vi "RT Main v1.9.vi"() -> ()   [LabVIEW 2021]
doc: "Changelog:\n\nv1.9:\n- Added a new shift register for \"clean resume\" which is reset when starting autocycle, and when performing a homing. It is set always after completing autocycle.\n\nv0.9:\n- Autocycle"
uses:
  Controls/Auto Delays.ctl
  Controls/DO 1.ctl
  Controls/Modbus Input.ctl
  support/Controls/General Para.ctl
  support/Controls/All Inputs.ctl
  Controls/DI 1.ctl
  Controls/DI 2.ctl
  support/Controls/Index Details.ctl
  support/Controls/Auto Stats.ctl
  Controls/Auto Times.ctl
  Global Variables/RT GV.vi
  support/Message Queue/Enqueue Message (Single).vi
  Global Variables/FPGA GV.vi
  <vilib>/Utility/error.llb/Error Cluster From Error Code.vi
  <vilib>/rvi/errors/niLvFpgaAdjustHostInterfaceError.vi
  Global Variables/Network Globals.vi
  <vilib>/FPGAPlugInAG/Dynamic/niLvFpga_Close_Dynamic.vi
  <vilib>/Modbus/master/Modbus Master.lvclass
  <vilib>/rvi/interface/nirviReadWriteControl/nirviReadWriteControl.xnode
  <vilib>/rvi/interface/nirviCloseFPGA/nirviCloseFPGA.xnode
  Controls/FPGA Ref.ctl
  support/Message Queue/Message Queue.lvlib
  NiFpgaLv.dll
  <vilib>/rvi/interface/Simulation/niFpgaSimulationCallBeginRW.vi
panel:
  in  "Auto Para":T1={"Agitator Delays"=[250, 350], "TF Delays"=[700, 800, 2], "Insertion Delays"=[100, 500], "Cutting Delays"=[300, 300, 100], "PF Delays"=[250, 30000], "Measur. Delays"=[500.0, 188.9, 1.0], "Reject Delays"=[500], "BF Delays"=[1000, 1000], "P&P Delays"=[1000]}
  in  "Stop Button 4":bool
  out "error out":errorcluster
  out "Wrong Message":string
  in  "Stop Button":bool
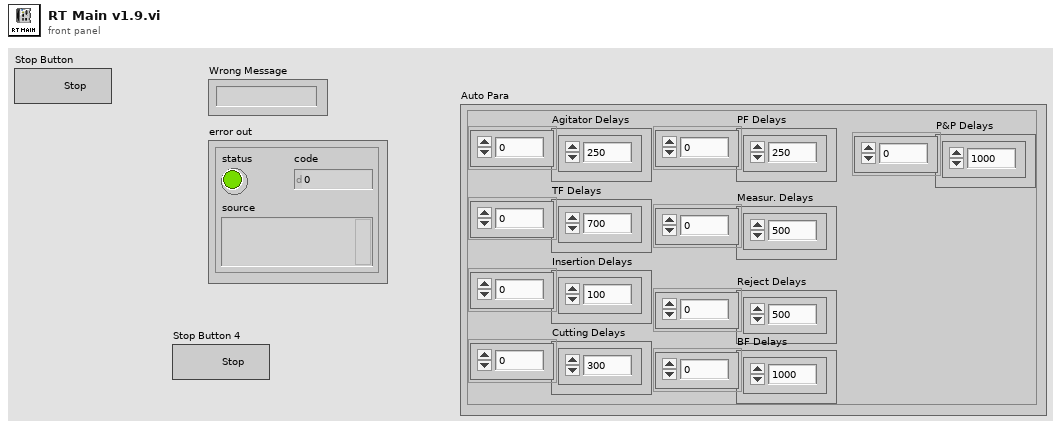
[diagram p1: front panel]
types:
  T1 = typedef "Auto Delays.ctl" = cluster{"Agitator Delays":u32[], "TF Delays":u32[], "Insertion Delays":u32[], "Cutting Delays":u32[], "PF Delays":u32[], "Measur. Delays":dbl[], "Reject Delays":u32[], "BF Delays":u32[], "P&P Delays":u32[]}
  T2 = typedef "FPGA Ref.ctl" = refnum<k20>
  T3 = typedef "DO 1.ctl" = cluster{"TL_Red":bool, "TL_Orange":bool, "TL_Green":bool, "TL_Buzzer":bool, "Vaccuum ON":bool, "Vaccuum OFF":bool, "Beckhoff Data":bool, "SOL_Singling":bool, "Bowl  Feeder_ ON 1":bool, "Buffer":bool, "SOL_Pick_Place_Vertical":bool, "SOL_Tube_Feed_Agitatator":bool, "SOL_Tube_Feed_Gating_CYL":bool, "SOL_Insertion _CYL":bool, "SOL_Insertion_Clamp_CYL":bool, "SOL_Cutting_CYL":bool, "SOL_Cutting_Clamp_CYL":bool, "SOL_Cutting_Foward_CYL":bool, "SOL_Measurement_CYL":bool, "SOL_Pick_Place_Rotary":bool, "SOL_Rejection CYL_1":bool, "SOL_Rejection CYL_2":bool, "SOL_Rejection CYL_3":bool, "SOL_Rejection CYL_4":bool, "Bowl  Feeder_ ON 2":bool, "Linear_Feeder 1":bool, "Linear_Feeder 2":bool, "Buffer 2":bool, "Buffer 3":bool, "Buffer 4":bool, "Buffer 5":bool, "Buffer 6":bool}
  T4 = typedef "Modbus Input.ctl" = cluster{"Maintenance Mode":bool, "Servo ON":bool, "Start":bool, "Stop":bool, "Reset Fault":bool, "Position Mode":bool, "Velocity Mode":bool, "Index":bool, "Start Index":bool, "Home":bool, "Start":bool, "Maintenance Position":i32, "Maintenance Hardware Torque":u16, "Maintenance Software Torque":u16, "Index Timeout":i16, "Index Position":i32, "Index Hardware Torque Limit":u16, "Index Software Torque Limit":u16, "Homing Timeout":i16, "Prehoming Position":i32, "Prehoming Hardware Torque Limit":u16, "Prehoming Software Torque Limit":u16, "Homing Position":i32, "Homing Hardware Torque Limit":u16, "Homing Software Torque Limit":u16}
  T5 = typedef "General Para.ctl" = cluster{"Max. Cons.":dbl, "Offset 1":dbl, "Offset 2":dbl, "Offset 3":dbl, "Offset 4":dbl, "OutputPause":dbl, "RejectPause":dbl, "IndexTimeout":dbl}
  T6 = typedef "All Inputs.ctl" = cluster{"DI 1":T7, "DI 2":T8, "IAS 1":dbl, "IAS 2":dbl, "IAS 3":dbl, "IAS 4":dbl, "DO 1":T3}
  T7 = typedef "DI 1.ctl" = cluster{"Machine_ON":bool, "E_stop ":bool, "SW_Pressure":bool, "SW_Start ":bool, "SW_Reset":bool, "SW_Stop":bool, "SW_Door":bool, "Buffer 1":bool, "Buffer 2":bool, "RS_Index_Stopper _Rear":bool, "RS_Singling_Rear":bool, "IPS_Index_Pallet_Sensor":bool, "PES_Index_Output_Part Sensor":bool, "Buffer 3":bool, "SW_Cutting_Station_Door":bool, "PES_BF_Pump_CNVR_Full_1":bool, "PES_BF_Pump_CNVR_Full_2":bool, "PES_BF_Pump_CNVR_Full_3":bool, "PES_BF_Pump_CNVR_Full_4":bool, "PES_PC_Pump Presence_1":bool, "PES_PC_Pump Presence_2":bool, "PES_PC_Pump Presence_3":bool, "PES_PC_Pump Presence_4":bool, "RS_Pick_Place_Vertical":bool, "Buffer 5":bool, "PES_TF_Low_Level":bool, "RS_Cutting_Rear1":bool, "RS_Cutting_Rear2":bool, "RS_Cutting_Rear3":bool, "RS_Cutting_Rear4":bool, "RS_Cutting_Forward_Rear":bool, "Buffer 11":bool}
  T8 = typedef "DI 2.ctl" = cluster{"RS_Agitatator_1_Rear":bool, "Buffer 1 ":bool, "RS_TF_Gating CYL_Rear":bool, "RS_Insertion_1_Rear":bool, "RS_Insertion_1_Front":bool, "RS_Insertion _2_Rear":bool, "RS_Insertion _2_Front":bool, "RS_Insertion _3_Rear":bool, "RS_Insertion _3_Front":bool, "RS_Insertion _4_Rear":bool, "RS_Insertion _4_Front":bool, "RS_Insertion_Clamp_CYL":bool, "RS_Cutting_Rear":bool, "RS_Clamping_Rear":bool, "RS_Measurement_Front":bool, "RS_Measurement_Rear":bool, "Buffer 2":bool, "Buffer 3":bool, "Buffer 4":bool, "RS_Rejection_1_Rear":bool, "RS_Rejection_2_Rear":bool, "RS_Rejection_3_Rear":bool, "RS_Rejection_4_Rear":bool, "Buffer 5":bool, "Buffer 6":bool, "LS_Rotary_P&P":bool, "Vaccum Components check":bool, "Buffer 9":bool, "Buffer 10":bool, "Buffer 11":bool, "Buffer 12":bool, "Buffer 13":bool}
  T9 = typedef "Index Details.ctl" = cluster{"Time (ms)":u32, "Waveform Graph":i16[]}
  T10 = cluster{T1, "Reject Pallets":cluster{"Reject 1":bool, "Reject 2":bool, "Reject 3":bool, "Reject 4":bool}}
  T11 = typedef "Auto Stats.ctl" = cluster{"Time-Stamp":timestamp, "Auto Times":T12, "Measurements":cluster{"1":dbl, "2":dbl, "3":dbl, "4":dbl}, "Outputs":cluster{"Good Parts":u32, "Reject Parts":u32}, "Cycle Time":dbl, "Remarks":string}
  T12 = typedef "Auto Times.ctl" = cluster{"Index Time":u32, "TF Time":u32, "Insertion Time":u32, "Cutting Time":u32, "PF Time":u32, "Meas. Time":u32, "Reject Time":u32, "P&P Time":u32}
  T13 = cluster{string, dbl, "cluster":cluster{"Auto Para":T1, "General Para":T5}}
  T14 = cluster{"TL_Red":bool, "TL_Orange":bool, "TL_Green":bool, "TL_Buzzer":bool, "Vaccuum ON":bool, "Vaccuum OFF":bool, "Beckhoff Data":bool, "SOL_Singling":bool, "Bowl Feeder_ ON1":bool, "Buffer 1":bool, "SOL_Pick_Place_Vertical":bool, "SOL_Tube_Feed_Agitatator":bool, "SOL_Tube_Feed_Gating_CYL":bool, "SOL_Insertion _CYL":bool, "SOL_Insertion_Clamp_CYL":bool, "SOL_Cutting_CYL":bool, "SOL_Cutting_Clamp_CYL":bool, "SOL_Insertion_Air_Nozzle":bool, "SOL_Measurement_CYL":bool, "SOL_Pick_Place_Rotary":bool, "SOL_Rejection CYL_1":bool, "SOL_Rejection CYL_2":bool, "SOL_Rejection CYL_3":bool, "SOL_Rejection CYL_4":bool, "Bowl Feeder_ON2":bool, "Linear Feeder 1":bool, "Linear Feeder 2":bool, "Buffer 2":bool, "Buffer 3":bool, "Buffer 4":bool, "Buffer 5":bool, "Buffer 6":bool}
  T15 = cluster{"Machine_ON":bool, "E_stop ":bool, "SW_Pressure":bool, "SW_Start ":bool, "SW_Reset":bool, "SW_Stop":bool, "SW_Door":bool, "Buffer 1":bool, "Buffer 2":bool, "RS_Index_Stopper _Rear":bool, "RS_Singling_Rear":bool, "PES_Index_Pallet_Sensor":bool, "PES_Index_Output_Part Sensor":bool, "Buffer 3":bool, "SW_Cutting_Station_Door":bool, "ICS_BF_Pump_CNVR_Full_1":bool, "ICS_BF_Pump_CNVR_Full_2":bool, "ICS_BF_Pump_CNVR_Full_3":bool, "ICS_BF_Pump_CNVR_Full_4":bool, "PES_PC_Pump Presence_1":bool, "PES_PC_Pump Presence_2":bool, "PES_PC_Pump Presence_3":bool, "PES_PC_Pump Presence_4":bool, "RS_Pick_Place_Vertical":bool, "Buffer 4":bool, "PES_TF_Low_Level":bool, "RS_Cutting_Rear 1":bool, "RS_Cutting_Rear 2":bool, "RS_Cutting_Rear 3":bool, "RS_Cutting_Rear 4":bool, "RS_Cutting_Forward_Rear":bool, "Buffer 10":bool}
  T16 = cluster{"RS_Agitatator_1_Rear ":bool, "Buffer 1 ":bool, "RS_TF_Gating CYL_Rear":bool, "RS_Insertion_1_Rear":bool, "RS_Insertion_1_Front":bool, "RS_Insertion _2_Rear":bool, "RS_Insertion _2_Front":bool, "RS_Insertion _3_Rear":bool, "RS_Insertion _3_Front":bool, "RS_Insertion _4_Rear":bool, "RS_Insertion _4_Front":bool, "RS_Insertion_Clamp_CYL":bool, "RS_Cutting_Rear":bool, "RS_Clamping_Rear":bool, "RS_Measurement_Front":bool, "RS_Measurement_Rear":bool, "Buffer 3":bool, "Buffer 4":bool, "Buffer 5":bool, "RS_Rejection_1_Rear":bool, "RS_Rejection_2_Rear":bool, "RS_Rejection_3_Rear":bool, "RS_Rejection_4_Rear":bool, "Buffer 6 ":bool, "Buffer 7 ":bool, "LS_Rotary_P&P":bool, "Vaccum Components check":bool, "Buffer 10 ":bool, "Buffer 11 ":bool, "Buffer 12 ":bool, "Buffer 13 ":bool, "Buffer 14":bool}
  T17 = cluster{"Array":string[][], "Machine Status":string}
  T18 = cluster{"Measurements":cluster{"1":dbl, "2":dbl, "3":dbl, "4":dbl}, "Reject Pallets":cluster{"Reject 1":bool, "Reject 2":bool, "Reject 3":bool, "Reject 4":bool}}
  T19 = cluster{"Auto Times":T12, "Results":cluster{"Measurements":cluster{"1":dbl, "2":dbl, "3":dbl, "4":dbl}, "Reject Pallets":cluster{"Reject 1":bool, "Reject 2":bool, "Reject 3":bool, "Reject 4":bool}}, "OutputCount":u32, "error out":errorcluster}
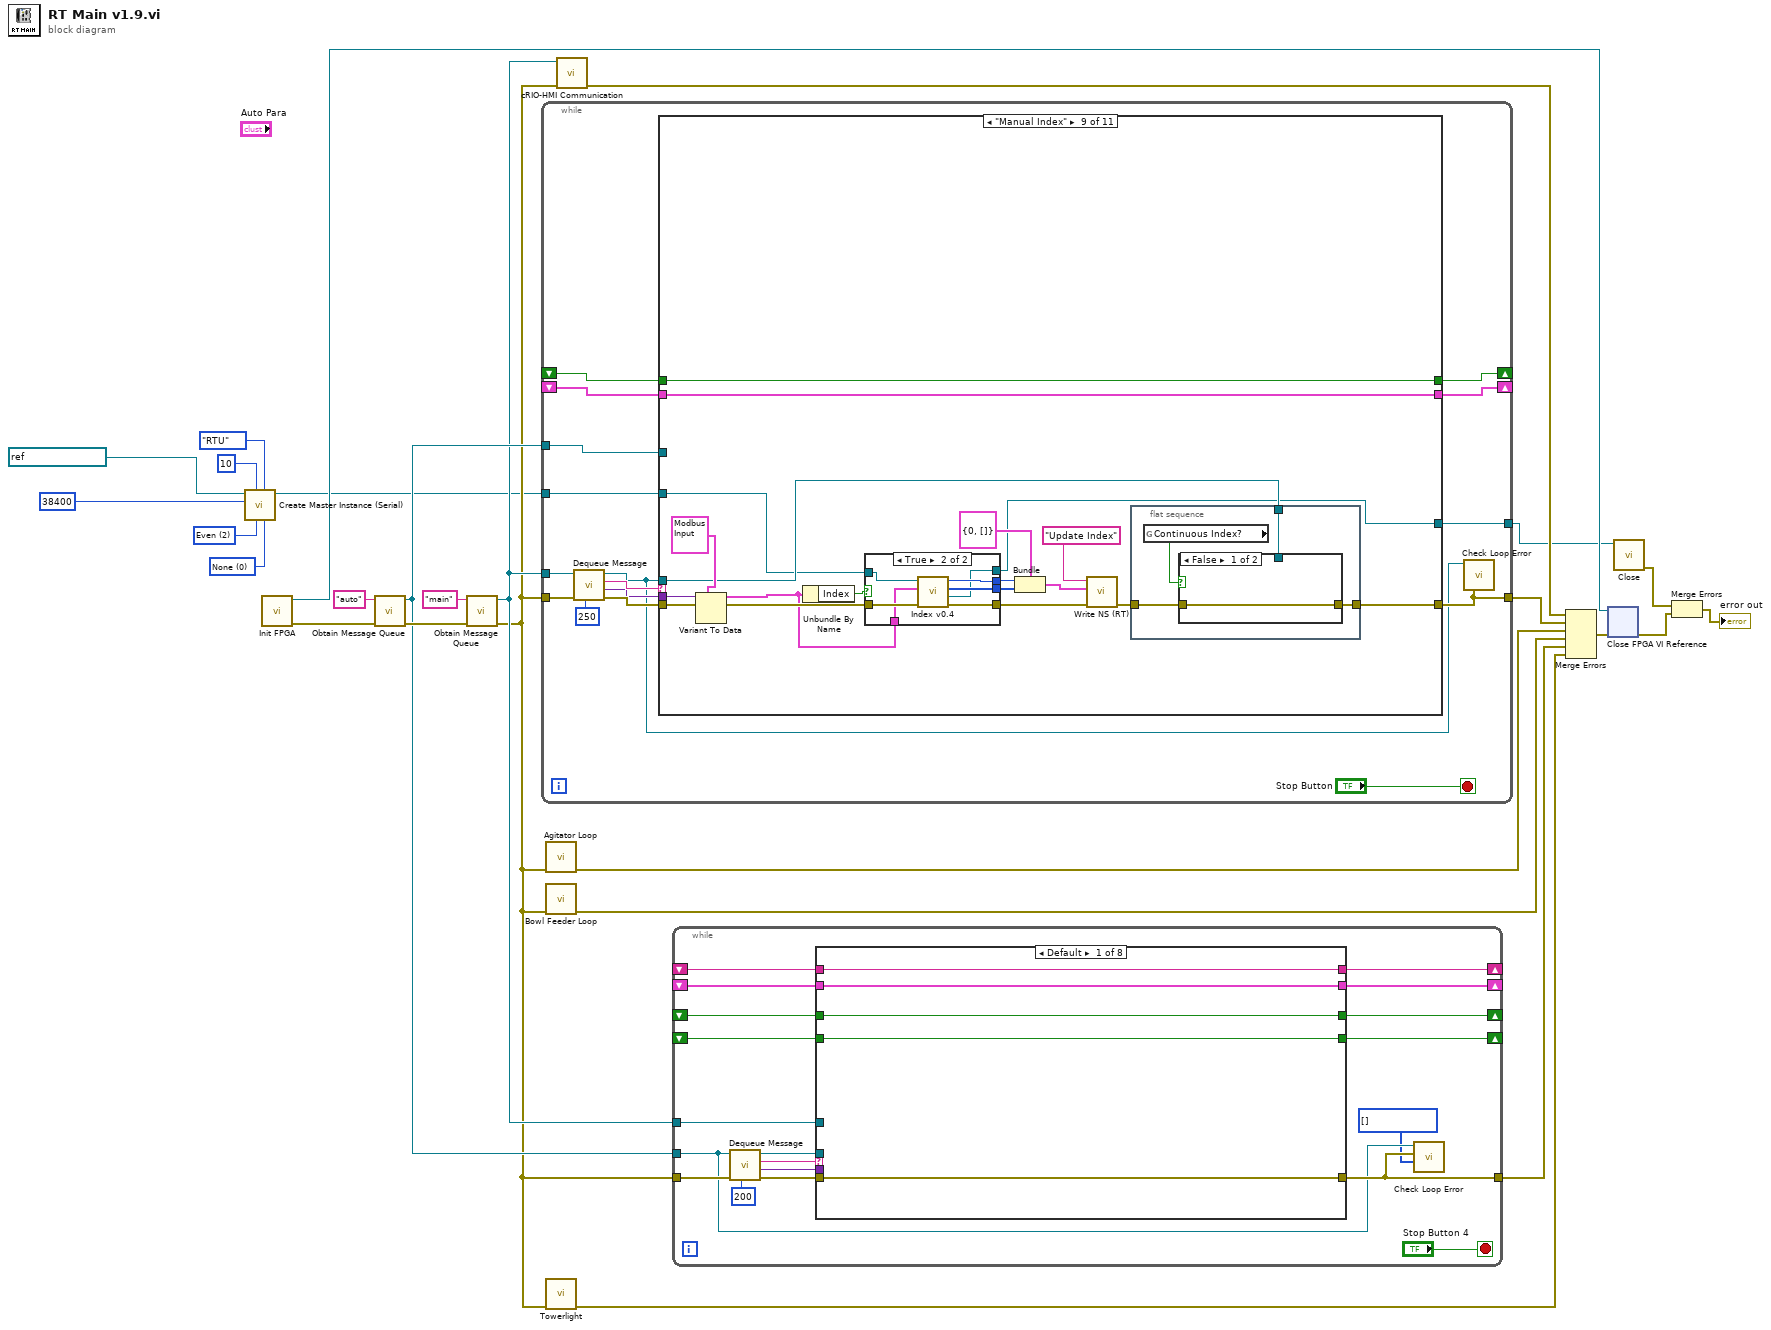
[diagram p0: block diagram]
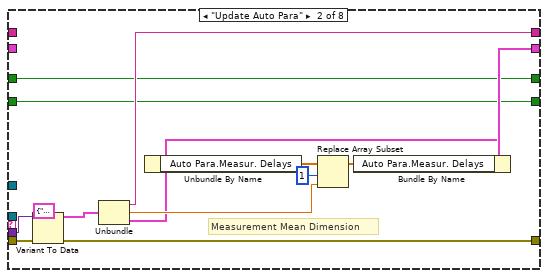
[diagram p2: hidden frame]
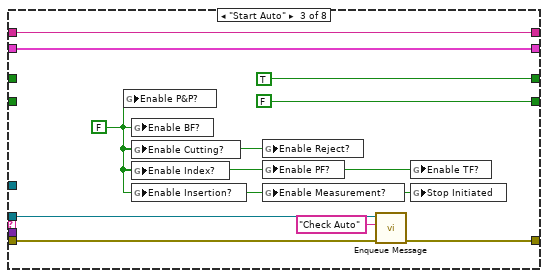
[diagram p3: hidden frame]
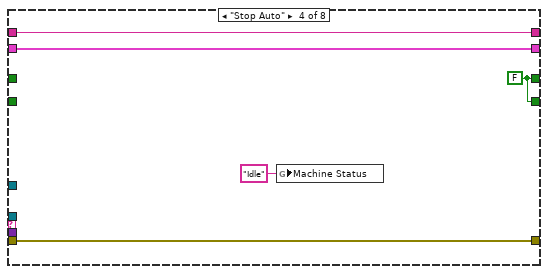
[diagram p4: hidden frame]
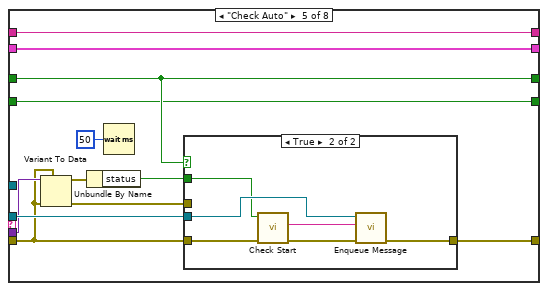
[diagram p5: hidden frame]
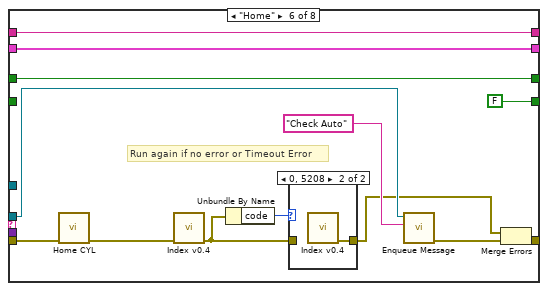
[diagram p7: hidden frame]
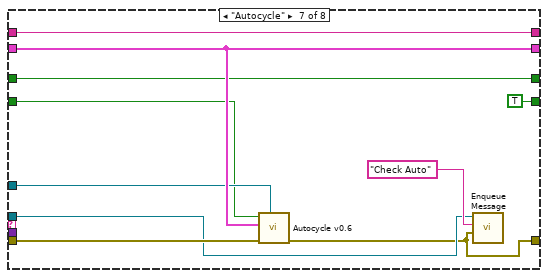
[diagram p9: hidden frame]
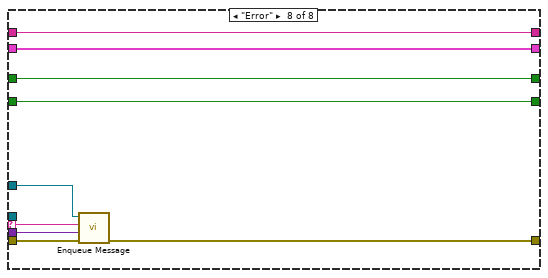
[diagram p10: hidden frame]
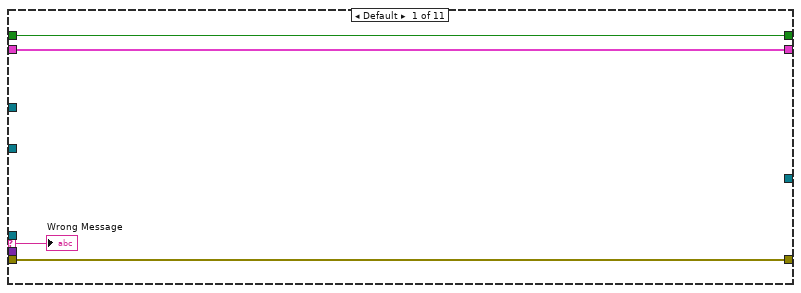
[diagram p11: hidden frame]
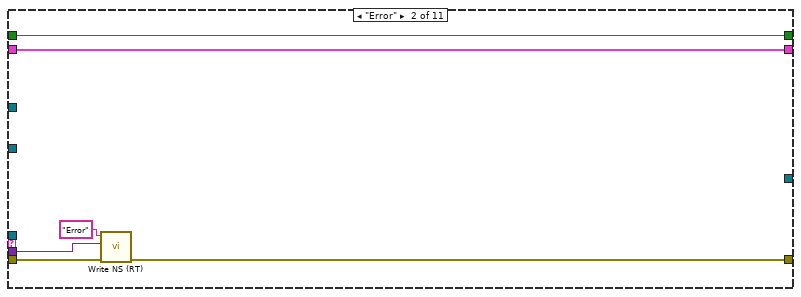
[diagram p12: hidden frame]
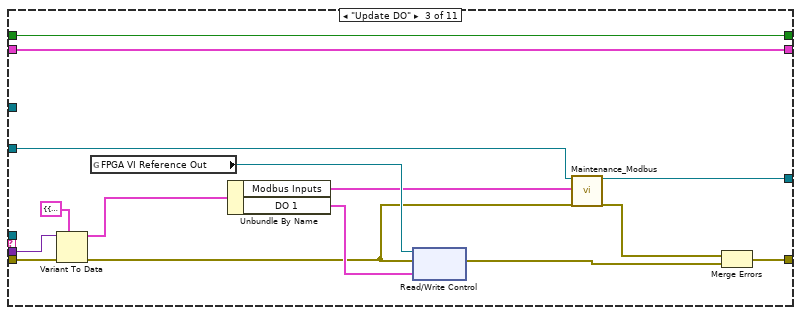
[diagram p13: hidden frame]
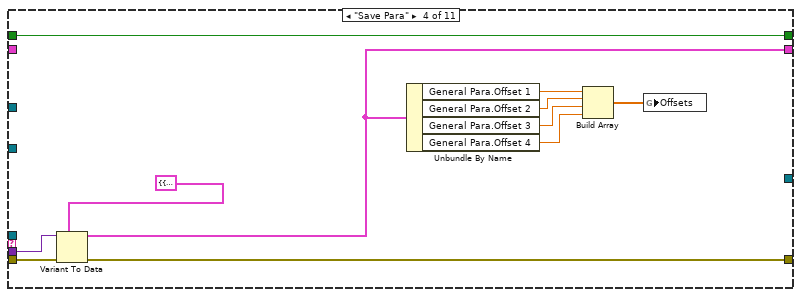
[diagram p14: hidden frame]
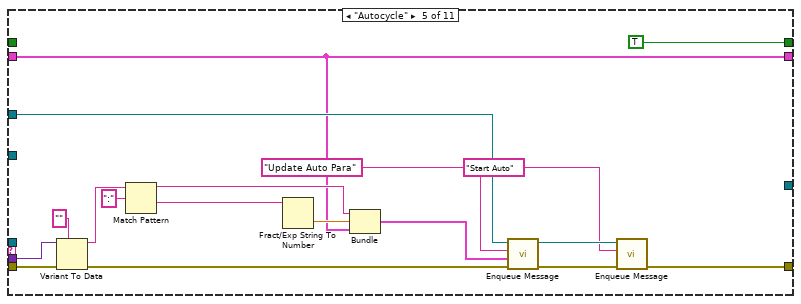
[diagram p15: hidden frame]
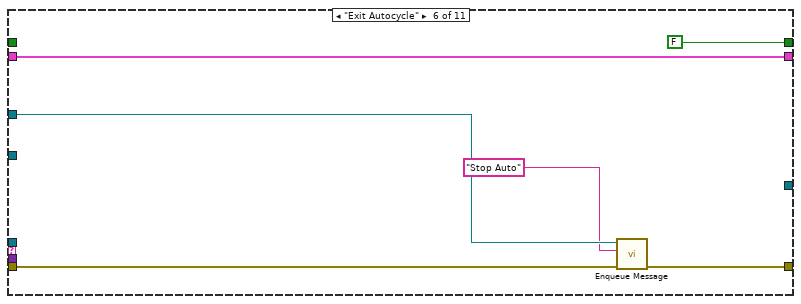
[diagram p16: hidden frame]
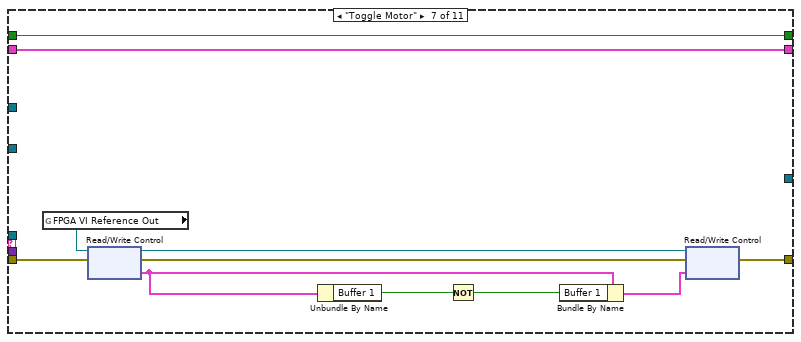
[diagram p17: hidden frame]
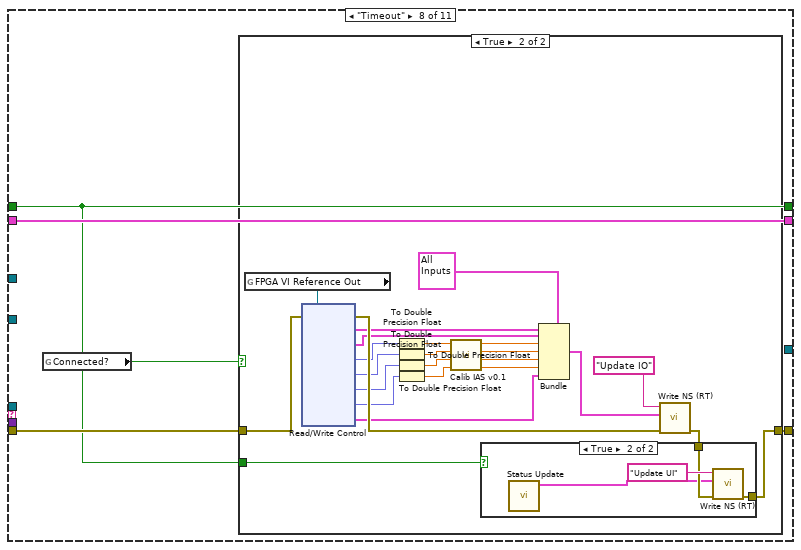
[diagram p18: hidden frame]
diagram:
  w6 = u16 0 items=["None", "XON/XOFF", "RTS/CTS", "XON/XOFF & RTS/CTS", "DTR/DSR", "XON/XOFF & DTR/DSR"] ("flow control (None)")
  w7 = u16 2 items=["None", "Odd", "Even"] ("parity (Even)")
  n1 = call <vilib>:"Create Master Instance (Serial).vi"("flow control (None)"=w6, "serial type"=enum16{"RTU", "ASCII"}."RTU", "parity (Even)"=w7, "unit ID"=u8 10, "baud rate (9600)"=u32 38400, "VISA resource name"=refnum<visa-resource-name> "ASRL1::INSTR") -> ("serial master instance"=w2:refnum<class "Modbus Master.lvclass">)  [unwired: 4 in, 1 out]
  n2 = call "Init FPGA.vi"() -> ("error out"=w17:errorcluster, "FPGA Ref Out"=w21:T2)  [unwired: 10 in]
  n3 = call "Obtain Message Queue.vi"("error in (no error)"=w17, "name"="auto") -> ("error out"=w16:errorcluster, "Message Queue"=w15:refnum<queue>)  [unwired: 8 in]
  n4 = call "Obtain Message Queue.vi"("error in (no error)"=w16, "name"="main") -> ("error out"=w13:errorcluster, "Message Queue"=w14:refnum<queue>)  [unwired: 8 in]
  n5 = while {
    tunnel: w13 -> [w41]
    tunnel: w14 -> [w40]
    tunnel: [w36] -> w26
    tunnel: w15 -> [w33]
    shift-right: [w31] -> _
    shift-left: _ -> [w32]
    shift-right: [w29] -> _
    shift-left: _ -> [w30]
    tunnel: w2 -> [w27]
    tunnel: [w28] -> w1
    stop <- "Stop Button" stop-if-true
    n6 = call "Dequeue Message.vi"("timeout"=250, "error in (no error)"=w41, "Message Queue"=w40) -> ("error out"=w39:errorcluster, "Message Data"=w37:variant, "Message"=w38:string, "dup Message Queue"=w35:refnum<queue>)  [unwired: 5 in]
    n7 = case shown="\"Manual Index\"" w38 {
      selector: w38 -> [w46 _ _ _ _ _ _ _ _ _ _]
      tunnel: w39 -> [w45 w51 w67 w78 w96 w102 w112 w117 w166 w204 w214]
      tunnel: w35 -> [_ _ _ _ _ _ _ _ w153 _ _]
      tunnel: w37 -> [_ w49 w66 w77 w95 _ _ _ w155 w203 w213]
      tunnel: [w45 w50 w55 w76 w82 w99 w110 w118 w159 w199 w210] -> w36
      tunnel: w33 -> [_ _ _ _ w88 w101 _ _ _ _ _]
      tunnel: w32 -> [w44 w52 w64 _ w85 w100 w104 w115 w156 w190 w209]
      tunnel: [w44 w52 w64 w73 w85 w100 w104 w115 w156 w190 w209] -> w31
      tunnel: w30 -> [w43 w47 w63 w75 _ _ w103 w114 w157 w187 w205]
      tunnel: [w43 w47 w63 w75 TRUE FALSE w103 w114 w157 w187 w205] -> w29
      tunnel: [_ _ w54 _ _ _ _ _ w150 w185 _] -> w28
      tunnel: w27 -> [_ _ w53 _ _ _ _ _ w151 w186 _]
      frame Default {
        "Wrong Message" <- w46
      }
      frame "Error" {
        n8 = call "Write NS (RT).vi"("error in (no error)"=w51, "Message Data"=w49, "Message"="Error") -> ("error out"=w50:errorcluster)  [unwired: 8 in]
      }
      frame "Update DO" {
        n9 = Variant To Data(error in=w67, type=cluster{"DO 1":T3, "Modbus Inputs":T4} {"DO 1"={"TL_Red"=FALSE, "TL_Orange"=FALSE, "TL_Green"=FALSE, "TL_Buzzer"=FALSE, "Vaccuum ON"=FALSE, "Vaccuum OFF"=FALSE, "Beckhoff Data"=FALSE, "SOL_Singling"=FALSE, "Bowl  Feeder_ ON 1"=FALSE, "Buffer"=FALSE, "SOL_Pick_Place_Vertical"=FALSE, "SOL_Tube_Feed_Agitatator"=FALSE, "SOL_Tube_Feed_Gating_CYL"=FALSE, "SOL_Insertion _CYL"=FALSE, "SOL_Insertion_Clamp_CYL"=FALSE, "SOL_Cutting_CYL"=FALSE, "SOL_Cutting_Clamp_CYL"=FALSE, "SOL_Cutting_Foward_CYL"=FALSE, "SOL_Measurement_CYL"=FALSE, "SOL_Pick_Place_Rotary"=FALSE, "SOL_Rejection CYL_1"=FALSE, "SOL_Rejection CYL_2"=FALSE, "SOL_Rejection CYL_3"=FALSE, "SOL_Rejection CYL_4"=FALSE, "Bowl  Feeder_ ON 2"=FALSE, "Linear_Feeder 1"=FALSE, "Linear_Feeder 2"=FALSE, "Buffer 2"=FALSE, "Buffer 3"=FALSE, "Buffer 4"=FALSE, "Buffer 5"=FALSE, "Buffer 6"=FALSE}, "Modbus Inputs"={"Maintenance Mode"=FALSE, "Servo ON"=FALSE, "Start"=FALSE, "Stop"=FALSE, "Reset Fault"=FALSE, "Position Mode"=FALSE, "Velocity Mode"=FALSE, "Index"=FALSE, "Start Index"=FALSE, "Home"=FALSE, "Start"=FALSE, "Maintenance Position"=0, "Maintenance Hardware Torque"=0, "Maintenance Software Torque"=0, "Index Timeout"=0, "Index Position"=0, "Index Hardware Torque Limit"=0, "Index Software Torque Limit"=0, "Homing Timeout"=0, "Prehoming Position"=0, "Prehoming Hardware Torque Limit"=0, "Prehoming Software Torque Limit"=0, "Homing Position"=0, "Homing Hardware Torque Limit"=0, "Homing Software Torque Limit"=0}}, Variant=w66) -> (data=w61:cluster{"DO 1":T3, "Modbus Inputs":T4}, error out=w58:errorcluster)
        n10 = global read "FPGA GV.vi" "FPGA VI Reference Out"() -> (w65:refnum<k20>)
        n11 = Unbundle By Name(w61) -> ("Modbus Inputs"=w59:T4, "DO 1"=w60:T3)
        n12 = xnode "Read/Write Control"("FPGA VI Reference In"=w65, "error in"=w58, "DO 1"=w60) -> ("error out"=w56:errorcluster)  [unwired: 1 out]
        n13 = call "Maintenance_Modbus.vi"("Modbus master in"=w53, "Modbus Inputs"=w59, "error in"=w58) -> ("Modbus master out"=w54:refnum<class "Modbus Master.lvclass">, "error out"=w57:errorcluster)  [unwired: 15 in]
        n14 = Merge Errors(w57, w56) -> (w55:errorcluster)
      }
      frame "Save Para" {
        n15 = Variant To Data(error in=w78, type=cluster{"Auto Para":T1, "General Para":T5} {"Auto Para"={"Agitator Delays"=[], "TF Delays"=[], "Insertion Delays"=[], "Cutting Delays"=[], "PF Delays"=[], "Measur. Delays"=[], "Reject Delays"=[], "BF Delays"=[], "P&P Delays"=[1000]}, "General Para"={"Max. Cons."=0.0, "Offset 1"=0.0, "Offset 2"=0.0, "Offset 3"=0.0, "Offset 4"=0.0, "OutputPause"=0.0, "RejectPause"=0.0, "IndexTimeout"=0.0}} ("cluster"), Variant=w77) -> (data=w73:cluster{"Auto Para":T1, "General Para":T5}, error out=w76:errorcluster)
        n16 = Unbundle By Name(w73) -> ("General Para.Offset 1"=w72:dbl, "General Para.Offset 2"=w71:dbl, "General Para.Offset 3"=w70:dbl, "General Para.Offset 4"=w69:dbl)
        n17 = Build Array(w72, w71, w70, w69) -> (w68:dbl[])
        n18 = global write "RT GV.vi" "Offsets"(w68) -> ()
      }
      frame "Autocycle" {
        n19 = Variant To Data(error in=w96, type="", Variant=w95) -> (data=w91:string, error out=w89:errorcluster)
        n20 = Match Pattern(string=w91, regular expression=":") -> (before substring=w87:string, after substring=w92:string)  [unwired: 1 in, 2 out]
        n21 = Fract/Exp String To Number(string=w92) -> (number=w86:dbl)  [unwired: 3 in, 1 out]
        n22 = Bundle(w87, w86, "cluster"=w85) -> (w84:T13)  [unwired: 1 in]
        n23 = call-poly "Enqueue Message.vi"("error in (no error)"=w89, "Message Data"=w84, "Message"="Update Auto Para", "Message Queue"=w88) -> ("error out"=w83:errorcluster, "dup Message Queue"=w81:refnum<queue>)  [unwired: 6 in]
        n24 = call-poly "Enqueue Message.vi"("error in (no error)"=w83, "Message"="Start Auto", "Message Queue"=w81) -> ("error out"=w82:errorcluster)  [unwired: 7 in, 1 out]
      }
      frame "Exit Autocycle" {
        n25 = call-poly "Enqueue Message.vi"("error in (no error)"=w102, "Message"="Stop Auto", "Message Queue"=w101) -> ("error out"=w99:errorcluster)  [unwired: 7 in, 1 out]
      }
      frame "Toggle Motor" {
        n26 = global read "FPGA GV.vi" "FPGA VI Reference Out"() -> (w113:refnum<k20>)
        n27 = xnode "Read/Write Control"("FPGA VI Reference In"=w113, "error in"=w112) -> ("FPGA VI Reference Out"=w109:refnum<k20>, "error out"=w111:errorcluster, "DO 1"=w107:T14)
        n28 = Unbundle By Name(w107) -> ("Buffer 1"=w108:bool)
        n29 = Not(x=w108) -> (.not. x?=w105:bool)
        n30 = Bundle By Name(cluster=w107, "Buffer 1"=w105) -> (w106:T14)
        n31 = xnode "Read/Write Control"("FPGA VI Reference In"=w109, "error in"=w111, "DO 1"=w106) -> ("error out"=w110:errorcluster)  [unwired: 1 out]
      }
      frame "Timeout" {
        n32 = global read "Network Globals.vi" "Connected?"() -> (w116:bool)
        n33 = case shown="True" w116 {
          tunnel: [w119 w122] -> w118
          tunnel: w117 -> [w119 w142]
          tunnel: w114 -> [_ w120]
          frame False {
          }
          frame True {
            n34 = global read "FPGA GV.vi" "FPGA VI Reference Out"() -> (w121:refnum<k20>)
            n35 = xnode "Read/Write Control"("FPGA VI Reference In"=w121, "error in"=w142) -> ("error out"=w141:errorcluster, "DI 1"=w140:T15, "DI 2"=w139:T16, "AI0"=w138:fxp<+/-,27,6>, "AI1"=w137:fxp<+/-,27,6>, "AI2"=w136:fxp<+/-,27,6>, "AI3"=w135:fxp<+/-,27,6>, "DO 1"=w132:T14)  [unwired: 1 out]
            n36 = To Double Precision Float(number=w138) -> (double precision float=w125:dbl)
            n37 = To Double Precision Float(number=w137) -> (double precision float=w127:dbl)
            n38 = To Double Precision Float(number=w136) -> (double precision float=w129:dbl)
            n39 = To Double Precision Float(number=w135) -> (double precision float=w131:dbl)
            n40 = call "Calib IAS v0.1.vi"("x 4"=w131, "x 3"=w129, "x 2"=w127, "x"=w125) -> ("y 4"=w130:dbl, "y 3"=w128:dbl, "y 2"=w126:dbl, "y 1"=w124:dbl)  [unwired: 2 in, 2 out]
            n41 = Bundle(cluster=T6 {"DI 1"={"Machine_ON"=FALSE, "E_stop "=FALSE, "SW_Pressure"=FALSE, "SW_Start "=FALSE, "SW_Reset"=FALSE, "SW_Stop"=FALSE, "SW_Door"=FALSE, "Buffer 1"=FALSE, "Buffer 2"=FALSE, "RS_Index_Stopper _Rear"=FALSE, "RS_Singling_Rear"=FALSE, "IPS_Index_Pallet_Sensor"=FALSE, "PES_Index_Output_Part Sensor"=FALSE, "Buffer 3"=FALSE, "SW_Cutting_Station_Door"=FALSE, "PES_BF_Pump_CNVR_Full_1"=FALSE, "PES_BF_Pump_CNVR_Full_2"=FALSE, "PES_BF_Pump_CNVR_Full_3"=FALSE, "PES_BF_Pump_CNVR_Full_4"=FALSE, "PES_PC_Pump Presence_1"=FALSE, "PES_PC_Pump Presence_2"=FALSE, "PES_PC_Pump Presence_3"=FALSE, "PES_PC_Pump Presence_4"=FALSE, "RS_Pick_Place_Vertical"=FALSE, "Buffer 5"=FALSE, "PES_TF_Low_Level"=FALSE, "RS_Cutting_Rear1"=FALSE, "RS_Cutting_Rear2"=FALSE, "RS_Cutting_Rear3"=FALSE, "RS_Cutting_Rear4"=FALSE, "RS_Cutting_Forward_Rear"=FALSE, "Buffer 11"=FALSE}, "DI 2"={"RS_Agitatator_1_Rear"=FALSE, "Buffer 1 "=FALSE, "RS_TF_Gating CYL_Rear"=FALSE, "RS_Insertion_1_Rear"=FALSE, "RS_Insertion_1_Front"=FALSE, "RS_Insertion _2_Rear"=FALSE, "RS_Insertion _2_Front"=FALSE, "RS_Insertion _3_Rear"=FALSE, "RS_Insertion _3_Front"=FALSE, "RS_Insertion _4_Rear"=FALSE, "RS_Insertion _4_Front"=FALSE, "RS_Insertion_Clamp_CYL"=FALSE, "RS_Cutting_Rear"=FALSE, "RS_Clamping_Rear"=FALSE, "RS_Measurement_Front"=FALSE, "RS_Measurement_Rear"=FALSE, "Buffer 2"=FALSE, "Buffer 3"=FALSE, "Buffer 4"=FALSE, "RS_Rejection_1_Rear"=FALSE, "RS_Rejection_2_Rear"=FALSE, "RS_Rejection_3_Rear"=FALSE, "RS_Rejection_4_Rear"=FALSE, "Buffer 5"=FALSE, "Buffer 6"=FALSE, "LS_Rotary_P&P"=FALSE, "Vaccum Components check"=FALSE, "Buffer 9"=FALSE, "Buffer 10"=FALSE, "Buffer 11"=FALSE, "Buffer 12"=FALSE, "Buffer 13"=FALSE}, "IAS 1"=0.0, "IAS 2"=0.0, "IAS 3"=0.0, "IAS 4"=0.0, "DO 1"={"TL_Red"=FALSE, "TL_Orange"=FALSE, "TL_Green"=FALSE, "TL_Buzzer"=FALSE, "Vaccuum ON"=FALSE, "Vaccuum OFF"=FALSE, "Beckhoff Data"=FALSE, "SOL_Singling"=FALSE, "Bowl  Feeder_ ON 1"=FALSE, "Buffer"=FALSE, "SOL_Pick_Place_Vertical"=FALSE, "SOL_Tube_Feed_Agitatator"=FALSE, "SOL_Tube_Feed_Gating_CYL"=FALSE, "SOL_Insertion _CYL"=FALSE, "SOL_Insertion_Clamp_CYL"=FALSE, "SOL_Cutting_CYL"=FALSE, "SOL_Cutting_Clamp_CYL"=FALSE, "SOL_Cutting_Foward_CYL"=FALSE, "SOL_Measurement_CYL"=FALSE, "SOL_Pick_Place_Rotary"=FALSE, "SOL_Rejection CYL_1"=FALSE, "SOL_Rejection CYL_2"=FALSE, "SOL_Rejection CYL_3"=FALSE, "SOL_Rejection CYL_4"=FALSE, "Bowl  Feeder_ ON 2"=FALSE, "Linear_Feeder 1"=FALSE, "Linear_Feeder 2"=FALSE, "Buffer 2"=FALSE, "Buffer 3"=FALSE, "Buffer 4"=FALSE, "Buffer 5"=FALSE, "Buffer 6"=FALSE}}, "DI 1"=w140, "DI 2"=w139, "IAS 1"=w124, "IAS 2"=w126, "IAS 3"=w128, "IAS 4"=w130, "DO 1"=w132) -> (w134:T6)
            n42 = call "Write NS (RT).vi"("error in (no error)"=w141, "Message Data"=w134, "Message"="Update IO") -> ("error out"=w123:errorcluster)  [unwired: 8 in]
            n43 = case shown="True" w120 {
              tunnel: w123 -> [w144 w147]
              tunnel: [w144 w146] -> w122
              frame False {
              }
              frame True {
                n44 = call "Status Update.vi"() -> ("Status Cluster"=w145:T17)  [unwired: 11 in]
                n45 = call "Write NS (RT).vi"("error in (no error)"=w147, "Message Data"=w145, "Message"="Update UI") -> ("error out"=w146:errorcluster)  [unwired: 8 in]
              }
            }
          }
        }
      }
      frame "Manual Index" {
        n46 = Variant To Data(type=T4 {"Maintenance Mode"=FALSE, "Servo ON"=FALSE, "Start"=FALSE, "Stop"=FALSE, "Reset Fault"=FALSE, "Position Mode"=FALSE, "Velocity Mode"=FALSE, "Index"=FALSE, "Start Index"=FALSE, "Home"=FALSE, "Start"=FALSE, "Maintenance Position"=0, "Maintenance Hardware Torque"=0, "Maintenance Software Torque"=0, "Index Timeout"=0, "Index Position"=0, "Index Hardware Torque Limit"=0, "Index Software Torque Limit"=0, "Homing Timeout"=0, "Prehoming Position"=0, "Prehoming Hardware Torque Limit"=0, "Prehoming Software Torque Limit"=0, "Homing Position"=0, "Homing Hardware Torque Limit"=0, "Homing Software Torque Limit"=0} ("Modbus Input"), Variant=w155) -> (data=w149:T4)  [unwired: 1 in, 1 out]
        n47 = Unbundle By Name(w149) -> ("Index"=w152:bool)
        n48 = case shown="True" w152 {
          tunnel: w166 -> [w168 w175]
          tunnel: [w168 w174] -> w164
          tunnel: [_ w173] -> w163
          tunnel: [_ w172] -> w162
          tunnel: w151 -> [w167 w171]
          tunnel: [w167 w170] -> w150
          tunnel: w149 -> [_ w169]
          frame False {
          }
          frame True {
            n49 = call "Index v0.4.vi"("error in (no error)"=w175, "Modbus Input"=w169, "Modbus master in"=w171) -> ("error out"=w174:errorcluster, "Modbus master out"=w170:refnum<class "Modbus Master.lvclass">, "Waveform Graph"=w172:i16[], "Index Time"=w173:u32)  [unwired: 4 in, 1 out]
          }
        }
        n50 = Bundle(cluster=T9 {"Time (ms)"=0, "Waveform Graph"=[]}, "Time (ms)"=w163, "Waveform Graph"=w162) -> (w161:T9)
        n51 = call "Write NS (RT).vi"("error in (no error)"=w164, "Message Data"=w161, "Message"="Update Index") -> ("error out"=w160:errorcluster)  [unwired: 8 in]
        n52 = flat-sequence {
          tunnel: w160 -> [w179]
          tunnel: [w178] -> w159
          tunnel: w153 -> [w176]
          frame #0 {
            n53 = global read "RT GV.vi" "Continuous Index?"() -> (w177:bool)
            n54 = case shown="False" w177 {
              tunnel: w179 -> [w180 w184]
              tunnel: [w180 w183] -> w178
              tunnel: w176 -> [_ w181]
              frame False {
              }
              frame True {
                n55 = call-poly "Enqueue Message.vi"("error in (no error)"=w184, "Message"="Manual Index", "Message Queue"=w181) -> ("error out"=w183:errorcluster)  [unwired: 7 in, 1 out]
              }
            }
          }
        }
      }
      frame "Manual Run" {
        n56 = Variant To Data(error in=w204, type=T10 {{"Agitator Delays"=[1000], "TF Delays"=[1000], "Insertion Delays"=[1000], "Cutting Delays"=[1000], "PF Delays"=[1000], "Measur. Delays"=[1000.0], "Reject Delays"=[1000], "BF Delays"=[1000], "P&P Delays"=[1000]}, "Reject Pallets"={"Reject 1"=FALSE, "Reject 2"=FALSE, "Reject 3"=FALSE, "Reject 4"=FALSE}}, Variant=w203) -> (data=w195:T10, error out=w202:errorcluster)
        n57 = Unbundle(w195) -> (w192:T1)  [unwired: 1 out]
        n58 = Unbundle By Name(w192) -> ("Agitator Delays"=w189:u32[], "BF Delays"=w188:u32[])
        n59 = call "Manual.vi"("error in"=w202, "Modbus master in"=w186, "Auto Delays"=w192) -> ("error out"=w194:errorcluster, "OutputCount"=w193:u32, "Results"=w191:T18, "Auto Times"=w198:T12, "Modbus master out"=w185:refnum<class "Modbus Master.lvclass">)  [unwired: 4 in]
        n60 = global write "RT GV.vi" "Agitator Delays"(w189) -> ()
        n61 = global write "RT GV.vi" "BF Delays"(w188) -> ()
        n62 = Bundle("Auto Times"=w198, "Results"=w191, "OutputCount"=w193, "error out"=w194) -> (w197:T19)  [unwired: 1 in]
        n63 = call "Write NS (RT).vi"("Message Data"=w197, "Message"="Manual Status") -> ("error out"=w200:errorcluster)  [unwired: 9 in]
        n64 = Merge Errors(w200) -> (w199:errorcluster)
      }
      frame "Log Cycle" {
        n65 = Variant To Data(error in=w214, type=T11 {"Time-Stamp"=timestamp(0 s since 1904-01-01), "Auto Times"={"Index Time"=0, "TF Time"=0, "Insertion Time"=0, "Cutting Time"=0, "PF Time"=0, "Meas. Time"=0, "Reject Time"=0, "P&P Time"=0}, "Measurements"={"1"=0.0, "2"=0.0, "3"=0.0, "4"=0.0}, "Outputs"={"Good Parts"=0, "Reject Parts"=0}, "Cycle Time"=0.0, "Remarks"=""} ("Auto Stats"), Variant=w213) -> (data=w206:T11, error out=w207:errorcluster)
        n66 = call "Write NS (RT).vi"("error in (no error)"=w207, "Message Data"=w206, "Message"="Autocycle Log") -> ("error out"=w211:errorcluster)  [unwired: 8 in]
        n67 = Merge Errors(w211) -> (w210:errorcluster)
      }
    }
    n68 = call "Check Loop Error.vi"("error to process"=w36, "Message Queue"=w35) -> ()  [unwired: 8 in, 2 out]
  }
  n69 = call "Agitator Loop.vi"("error in (no error)"=w13) -> ("error out"=w23:errorcluster)  [unwired: 10 in]
  n70 = call "Bowl Feeder Loop.vi"("error in (no error)"=w13) -> ("error out"=w22:errorcluster)  [unwired: 10 in]
  n71 = call "Towerlight.vi"("error in (no error)"=w13) -> ("error out"=w12:errorcluster)  [unwired: 10 in]
  n72 = call "cRIO-HMI Communication.vi"("error in (no error)"=w13, "Message Queue"=w14) -> ("error out"=w25:errorcluster)  [unwired: 9 in]
  n73 = while {
    tunnel: w13 -> [w231]
    tunnel: [w229] -> w20
    tunnel: w15 -> [w221]
    shift-right: [w225] -> _
    shift-left: _ -> [w224]
    shift-right: [w223] -> _
    shift-left: _ -> [w222]
    shift-right: [w220] -> _
    shift-left: _ -> [w219]
    tunnel: w14 -> [w218]
    shift-right: [w215] -> _
    shift-left: _ -> [w216]
    stop <- "Stop Button 4" stop-if-true
    n74 = call "Dequeue Message.vi"("timeout"=200, "error in (no error)"=w231, "Message Queue"=w221) -> ("error out"=w230:errorcluster, "Message Data"=w226:variant, "Message"=w227:string, "dup Message Queue"=w228:refnum<queue>)  [unwired: 5 in]
    n75 = case shown="Default" w227 {
      selector: w227 -> [_ _ _ _ _ _ _ w316]
      tunnel: w230 -> [w238 w252 w258 w264 w270 w295 w310 w314]
      tunnel: [w238 w251 w257 w264 w276 w289 w303 w313] -> w229
      tunnel: w228 -> [_ _ w256 _ w275 w290 w304 _]
      tunnel: w226 -> [_ w250 _ _ w272 _ _ w315]
      tunnel: [w237 w248 w261 w266 w278 w298 w309 w319] -> w225
      tunnel: w224 -> [w237 _ w261 w266 w278 w298 w309 w319]
      tunnel: [w236 w243 w260 w265 w277 w297 w308 w318] -> w223
      tunnel: w222 -> [w236 _ w260 w265 w277 w297 w308 w318]
      tunnel: [w235 w242 TRUE w262 w274 w296 w306 w317] -> w220
      tunnel: w219 -> [w235 w242 _ _ w274 w296 w306 w317]
      tunnel: w218 -> [_ _ _ _ _ _ w307 w312]
      tunnel: w216 -> [w234 w239 _ _ w267 _ w302 w311]
      tunnel: [w234 w239 FALSE w262 w267 FALSE TRUE w311] -> w215
      frame Default {
      }
      frame "Update Auto Para" {
        # "Measurement Mean Dimension"
        n76 = Variant To Data(error in=w252, type=T13 {"", 0.0, "cluster"={"Auto Para"={"Agitator Delays"=[], "TF Delays"=[], "Insertion Delays"=[], "Cutting Delays"=[], "PF Delays"=[], "Measur. Delays"=[], "Reject Delays"=[], "BF Delays"=[], "P&P Delays"=[1000]}, "General Para"={"Max. Cons."=0.0, "Offset 1"=0.0, "Offset 2"=0.0, "Offset 3"=0.0, "Offset 4"=0.0, "OutputPause"=0.0, "RejectPause"=0.0, "IndexTimeout"=0.0}}} ("cluster"), Variant=w250) -> (data=w249:T13, error out=w251:errorcluster)
        n77 = Unbundle(w249) -> (w248:string, w245:dbl, "cluster"=w241:cluster{"Auto Para":T1, "General Para":T5})
        n78 = Unbundle By Name(w241) -> ("Auto Para.Measur. Delays"=w247:dbl[])
        n79 = Replace Array Subset(array=w247, new element=w245, index=1) -> (w244:dbl[])
        n80 = Bundle By Name(cluster=w241, "Auto Para.Measur. Delays"=w244) -> (w243:cluster{"Auto Para":T1, "General Para":T5})
      }
      frame "Start Auto" {
        w253 = FALSE ("Enable BF?")
        n81 = global write "RT GV.vi" "Enable P&P?"(w253) -> ()
        n82 = global write "RT GV.vi" "Enable BF?"(w253) -> ()
        n83 = global write "RT GV.vi" "Enable Cutting?"(w253) -> ()
        n84 = global write "RT GV.vi" "Enable Index?"(w253) -> ()
        n85 = global write "RT GV.vi" "Enable Insertion?"(w253) -> ()
        n86 = global write "RT GV.vi" "Enable Reject?"(w253) -> ()
        n87 = global write "RT GV.vi" "Enable PF?"(w253) -> ()
        n88 = global write "RT GV.vi" "Enable Measurement?"(w253) -> ()
        n89 = call-poly "Enqueue Message.vi"("error in (no error)"=w258, "Message"="Check Auto", "Message Queue"=w256) -> ("error out"=w257:errorcluster)  [unwired: 7 in, 1 out]
        n90 = global write "RT GV.vi" "Enable TF?"(w253) -> ()
        n91 = global write "RT GV.vi" "Stop Initiated"(w253) -> ()
      }
      frame "Stop Auto" {
        w262 = FALSE
        n92 = global write "RT GV.vi" "Machine Status"("Idle" ("Machine Status")) -> ()
      }
      frame "Check Auto" {
        n93 = Variant To Data(error in=w270, type=w270, Variant=w272) -> (data=w269:errorcluster, error out=w271:errorcluster)
        n94 = Unbundle By Name(w269) -> ("status"=w268:bool)
        n95 = Wait (ms)(milliseconds to wait=u32 50) -> ()  [unwired: 1 out]
        n96 = case shown="True" w274 {
          tunnel: [w279 w285] -> w276
          tunnel: w275 -> [_ w281]
          tunnel: w270 -> [w279 w284]
          tunnel: w271 -> [_ _]
          tunnel: w268 -> [_ w280]
          frame False {
          }
          frame True {
            n97 = call "Check Start.vi"("error in"=w284, "Error Stop?"=w280) -> ("error out"=w283:errorcluster, "Message"=w282:string)  [unwired: 8 in]
            n98 = call-poly "Enqueue Message.vi"("error in (no error)"=w283, "Message"=w282, "Message Queue"=w281) -> ("error out"=w285:errorcluster)  [unwired: 7 in, 1 out]
          }
        }
      }
      frame "Home" {
        # "Run again if no error or Timeout Error"
        n99 = call "Home CYL.vi"("error in"=w295) -> ("error out"=w287:errorcluster)  [unwired: 10 in]
        n100 = call "Index v0.4.vi"("error in (no error)"=w287) -> ("error out"=w293:errorcluster)  [unwired: 6 in, 4 out]
        n101 = Unbundle By Name(w293) -> ("code"=w294:i32)
        n102 = case shown="0, 5208" w294 {
          tunnel: [w299 w300] -> w288
          tunnel: w293 -> [w299 _]
          frame Default {
          }
          frame 0, 5208 {
            n103 = call "Index v0.4.vi"() -> ("error out"=w300:errorcluster)  [unwired: 7 in, 4 out]
          }
        }
        n104 = call-poly "Enqueue Message.vi"("Message"="Check Auto", "Message Queue"=w290) -> ("error out"=w291:errorcluster)  [unwired: 8 in, 1 out]
        n105 = Merge Errors(w288, w291) -> (w289:errorcluster)
      }
      frame "Autocycle" {
        n106 = call "Autocycle v0.6.vi"("Message Queue"=w307, "error in"=w310, "All Para"=w308, "CleanResume?"=w302) -> ("error out"=w303:errorcluster)  [unwired: 7 in]
        n107 = call-poly "Enqueue Message.vi"("Message Data"=w303, "Message"="Check Auto", "Message Queue"=w304) -> ()  [unwired: 7 in, 2 out]
      }
      frame "Error" {
        n108 = call-poly "Enqueue Message.vi"("error in (no error)"=w314, "Message Data"=w315, "Message"=w316, "Message Queue"=w312) -> ("error out"=w313:errorcluster)  [unwired: 6 in, 1 out]
      }
    }
    n109 = call "Check Loop Error.vi"("Ignore Errors"=i32[] [], "error to process"=w229, "Message Queue"=w221) -> ()  [unwired: 7 in, 2 out]
  }
  n110 = Merge Errors(w25, w26, w23, w22, w20, w12) -> (w24:errorcluster)
  n111 = xnode ("Close FPGA VI Reference")("FPGA VI Reference In"=w21, "error in"=w24) -> ("error out"=w3:errorcluster)
  n112 = call-dynamic "Close.vi"("Modbus master in"=w1) -> ("error out"=w4:errorcluster)  [unwired: 10 in]
  n113 = Merge Errors(w4, w3) -> (→"error out":errorcluster)
